vi "Register for Abort Event.vi"(8 "error in (no error)":errorcluster, 10 "Abort User Event":refnum<user-event>, 11 "Slave Test Runner In":refnum<class "Slave Test Runner.lvclass">) -> (0 "error out":errorcluster, 3 "Slave Test Runner Out":refnum<class "Slave Test Runner.lvclass">)   [LabVIEW 2020, in "Slave Test Runner.lvclass"]
uses:
  Slave Test Runner.lvclass
  Slave Test Runner.lvclass/Slave Test Runner.ctl
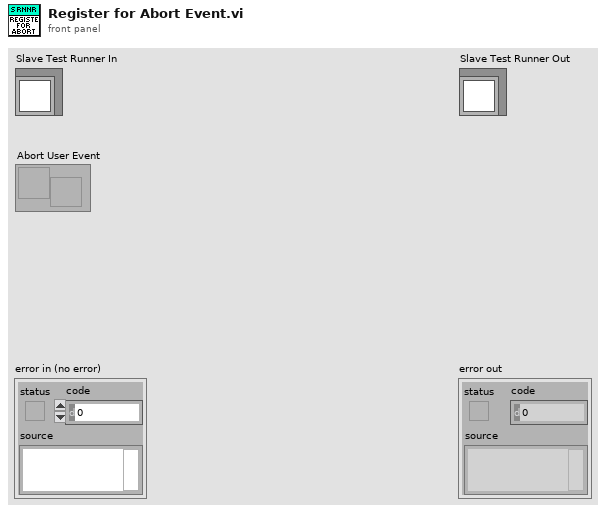
[diagram p1: front panel]
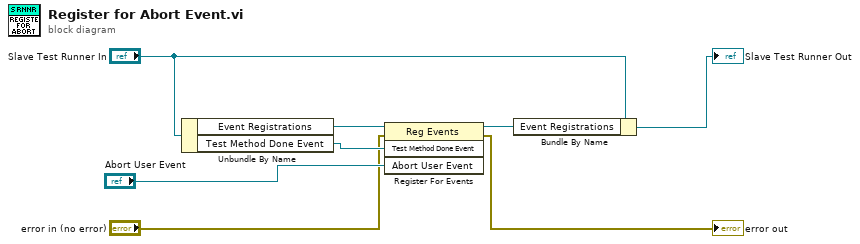
[diagram p0: block diagram]
diagram:
  n1 = Unbundle By Name("Slave Test Runner In") -> ("Event Registrations"=w4:refnum<event-registration>, "Test Method Done Event"=w6:refnum<user-event>)
  n2 = register-events(reference=w4, error in="error in (no error)", w6, "Abort User Event") -> (reference out=w3:refnum<event-registration>, error out=→"error out":errorcluster)
  n3 = Bundle By Name(cluster="Slave Test Runner In", "Event Registrations"=w3) -> (→"Slave Test Runner Out":refnum<class "Slave Test Runner.lvclass">)
